vi "NI VeriStand - Get Custom Device Channel Data.vi"(8 "error in (no error)":errorcluster, 11 "Channel Ref in":T3 format="%.0x") -> (0 "error out":errorcluster, 1 "Channel":T1, 2 "Channel Name":string, 3 "Channel Ref out":T3 format="%.0x", 4 "Found":bool, 5 "GUID":string)   [LabVIEW 2019, in "Custom Device API.lvlib"]
doc: "Returns information about the channel specified by <B>Channel Ref in</B>."
uses:
  Custom Device API.lvlib
  Custom Device Item Ref.ctl
  Custom Device Channel.ctl
  Custom Device Channel Type.ctl
  Custom Device Offline Path.vi
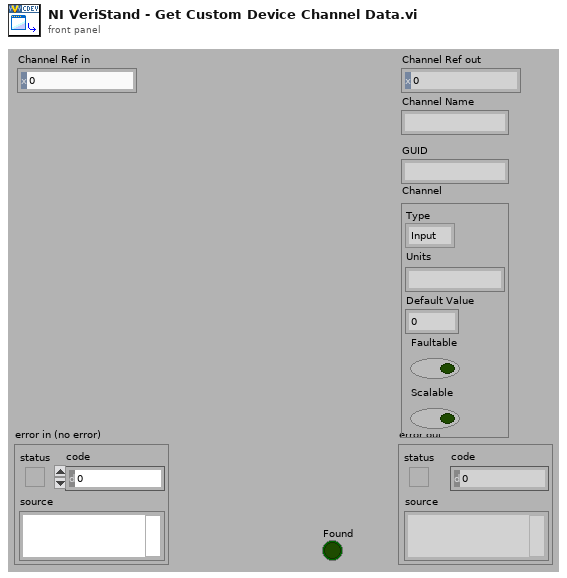
[diagram p1: front panel]
types:
  T1 = typedef "Custom Device API.lvlib/Custom Device Channel.ctl" = cluster{"Type":T2, "Units":string, "Default Value":dbl, "Faultable":bool, "Scalable":bool}
  T2 = typedef "Custom Device API.lvlib/Custom Device Channel Type.ctl" = enum16{"Input", "Output"}
  T3 = typedef "Custom Device API.lvlib/Custom Device Item Ref.ctl" = u64
  T4 = typedef "Custom Devices Storage.lvlib/Custom Device Channel.ctl" = cluster{"Type":T5, "Units":string, "Default Value":dbl, "Faultable":bool, "Scalable":bool}
  T5 = typedef "Custom Devices Storage.lvlib/Custom Device Channel Type.ctl" = enum16{"Input", "Output"}
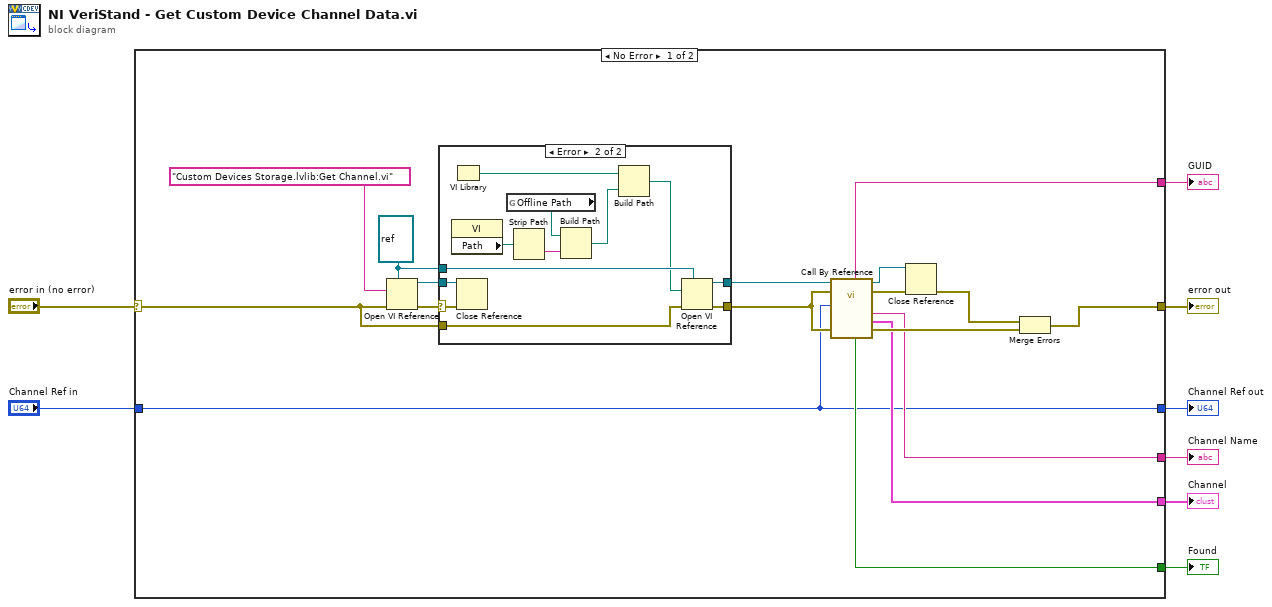
[diagram p0: block diagram]
diagram:
  n1 = case shown="No Error" "error in (no error)" {
    selector: "error in (no error)" -> [w18 w41]
    tunnel: "Channel Ref in" -> [w17 w40]
    tunnel: [w17 w40] -> w7
    tunnel: [w24 _] -> w6
    tunnel: [w23 _] -> w5
    tunnel: [w22 w41] -> w4
    tunnel: [w21 _] -> w3
    tunnel: [w20 _] -> w2
    frame No Error {
      w11 = refnum<vi> refnum ("type specifier VI Refnum (for type only)")
      n2 = Open VI Reference(type specifier VI Refnum (for type only)=w11, vi path="Custom Devices Storage.lvlib:Get Channel.vi", error in (no error)=w18) -> (vi reference=w12:refnum<vi>, error out=w13:errorcluster)  [unwired: 3 out]
      n3 = case shown="Error" w13 {
        selector: w13 -> [w26 w36]
        tunnel: w11 -> [_ w38]
        tunnel: w12 -> [w27 w37]
        tunnel: [w27 w35] -> w15
        tunnel: [w26 w34] -> w19
        tunnel: w18 -> [_ w39]
        frame No Error {
        }
        frame Error {
          n4 = property class="VI"() -> ("Path"=w29:path)  [unwired: 2 in, 2 out]
          n5 = VI Library() -> (path=w33:path)
          n6 = Close Reference(reference=w37, error in (no error)=w36) -> ()  [unwired: 1 out]
          n7 = global read "Custom Device Offline Path.vi" "Offline Path"() -> (w30:path)
          n8 = Strip Path(path=w29) -> (name=w28:string)  [unwired: 1 out]
          n9 = Build Path(base path=w30, name or relative path=w28) -> (appended path=w32:path)
          n10 = Build Path(base path=w33, name or relative path=w32) -> (appended path=w31:path)
          n11 = Open VI Reference(type specifier VI Refnum (for type only)=w38, vi path=w31, error in (no error)=w39) -> (vi reference=w35:refnum<vi>, error out=w34:errorcluster)  [unwired: 3 out]
        }
      }
      n12 = call-by-ref "?"(reference=w15, error in=w19, 8:"error in (no error)"=w19, "Channel Ref in"=w17) -> (reference out=w9:refnum<vi>, error out=w16:errorcluster, 0:"error out"=w25:errorcluster, "Channel"=w21:T4, "Channel Name"=w24:string, "Found"=w23:bool, "GUID"=w20:string)  [unwired: 4 in, 1 out]
      n13 = Close Reference(reference=w9, error in (no error)=w16) -> (error out=w10:errorcluster)
      n14 = Merge Errors(w10, w25) -> (w22:errorcluster)
    }
    frame Error {
    }
  }
  "Channel Ref out" <- w7
  "error out" <- w4
  "Channel" <- w3
  "Found" <- w5
  "GUID" <- w2
  "Channel Name" <- w6
